vi "Z Aux Direct Move Circ2.vi"(6 "fend2":sgl, 7 "fend1":sgl, 8 "error in (no error)":errorcluster caption="错误输入（无错误）", 9 "fmid2":sgl, 10 "fmid1":sgl, 11 "handle":u32) -> (0 "error out":errorcluster caption="错误输出", 2 "function return":i32, 3 "handle out":u32)   [LabVIEW 2015, in "zauxdll.lvlib"]
doc: "int32 __stdcall ZAux_Direct_MoveCirc2(ZMC_HANDLE handle, float fmid1, float fmid2, float fend1, float fend2);"
uses:
  zauxdll.lvlib
  zauxdll.dll
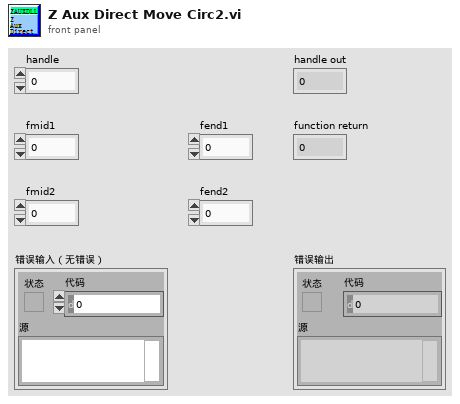
[diagram p1: front panel]
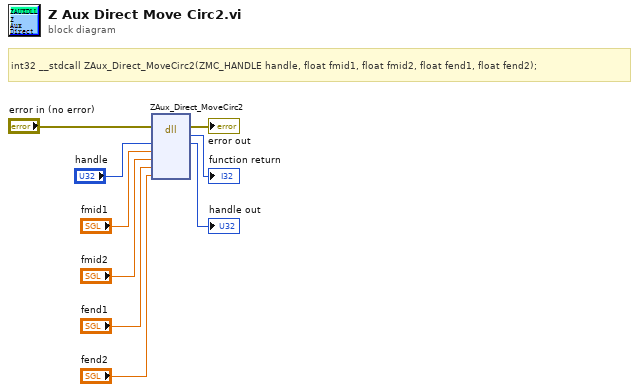
[diagram p0: block diagram]
diagram:
  # "int32 __stdcall ZAux_Direct_MoveCirc2(ZMC_HANDLE handle, float fmid1, float fmid2, float fend1, float fend2);"
  n1 = dll-call lib="C:/Users/VIC/Desktop/GOGORO_Oringnal - Panasonic/system/LLB/zmotion/zaux/zauxdll.*" fn="ZAux_Direct_MoveCirc2"(error in="error in (no error)", "handle"="handle", "fmid1"="fmid1", "fmid2"="fmid2", "fend1"="fend1", "fend2"="fend2") -> (error out=→"error out":errorcluster, →"function return":i32, "handle"=→"handle out":u32)  [unwired: 6 in, 1 out]
